vi "calibrate.vi"(8 "error in (no error)":errorcluster, 10 "device (1)":i32=1, 11 "Handle in":i64) -> (0 "error out":errorcluster, 2 "Return (<0 is error)":i32, 3 "Handle out":i64)   [LabVIEW 2016, in "OSB_uMp_library.lvlib"]
doc: "Sends calibrate command to uMp.\n\n!!! Ensure working area is clear before using this VI!!!\nuMp will move over its full range"
uses:
  OSB_uMp_library.lvlib
  ump.dll
panel:
  # "By Stuart Box at OxSyBio Ltd, 2017\n\nThis software is provided WITHOUT ANY WARRANTY; without even the implied warranty of MERCHANTABILITY or FITNESS FOR A PARTICULAR PURPOSE.\n\ninfo@oxsybio.com\n\nOxSyBio Ltd, The Walbrook Building, 25 Walbrook, London, EC4N 8AF"
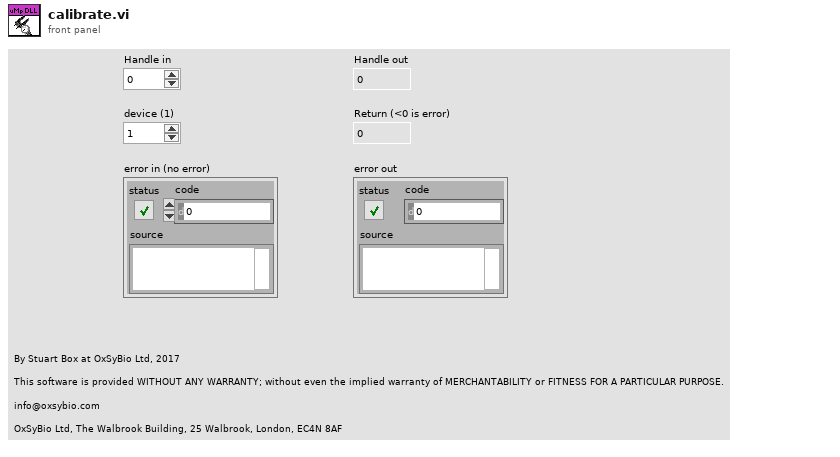
[diagram p1: front panel]
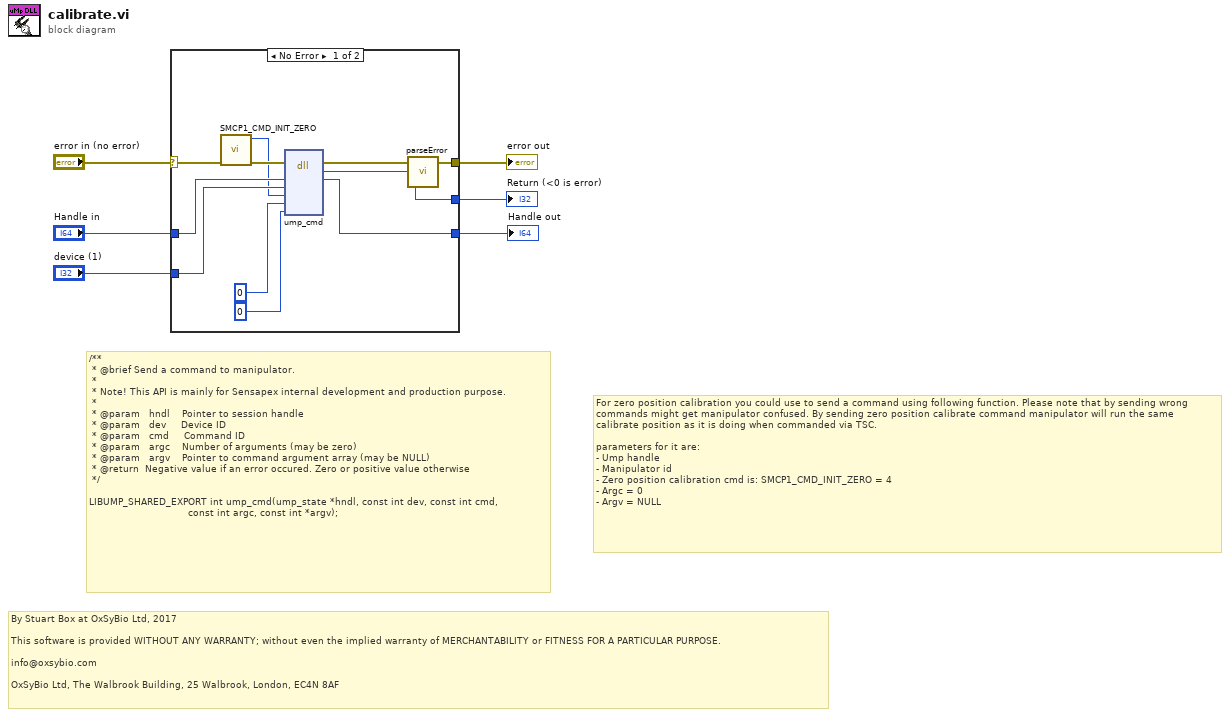
[diagram p0: block diagram]
diagram:
  # "By Stuart Box at OxSyBio Ltd, 2017\n\nThis software is provided WITHOUT ANY WARRANTY; without even the implied warranty of MERCHANTABILITY or FITNESS FOR A PARTICULAR PURPOSE.\n\ninfo@oxsybio.com\n\nOxSyBio Ltd, The Walbrook Building, 25 Walbrook, London, EC4N 8AF"
  # "For zero position calibration you could use to send a command using following function. Please note that by sending wrong commands might get manipulator confused. By sending zero position calibrate command manipulator will run the same calibrate position as it is doing when commanded via TSC.\n\nparameters for it are:\n-\tUmp handle\n-\tManipulator id\n-\tZero position calibration cmd is: SMCP1_CMD_INIT_ZERO = 4\n-\tArgc = 0\n-\tArgv = NULL"
  # "/**\n * @brief Send a command to manipulator.\n *\n * Note! This API is mainly for Sensapex internal development and production purpose.\n *\n * @param   hndl    Pointer to session handle\n * @param   dev     Device ID\n * @param   cmd     Command ID\n * @param   argc    Number of arguments (may be zero)\n * @param   argv    Pointer to command argument array (may be NULL)\n * @return  Negative value if an error occured. Zero or positive value otherwise\n */\n\nLIBUMP_SHARED_EXPORT int ump_cmd(ump_state *hndl, const int dev, const int cmd,\n                                 const int argc, const int *argv);"
  n1 = case shown="No Error" "error in (no error)" {
    selector: "error in (no error)" -> [w12 w19]
    tunnel: "Handle in" -> [w17 w18]
    tunnel: [w8 w19] -> w5
    tunnel: "device (1)" -> [w16 _]
    tunnel: [w7 _] -> w3
    tunnel: [w15 w18] -> w2
    frame No Error {
      n2 = call "SMCP1_CMD_INIT_ZERO.vi"("Error In"=w12) -> ("Error Out"=w11:errorcluster, "SMCP1_CMD_INIT_ZERO"=w10:i32)  [unwired: 9 in]
      n3 = dll-call lib="C:/Users/Stu/Desktop/OSB LabVIEW uMp/uMp_library/ump.dll" fn="ump_cmd"(error in=w11, "handle"=w17, "device"=w16, "command"=w10, "argc"=0, "argv"=0) -> (error out=w9:errorcluster, "return"=w7:i32, "handle"=w15:i64)  [unwired: 6 in, 1 out]
      n4 = call "parseError.vi"("Error In"=w9, "ump dll return value (<0 is error)"=w7) -> ("Error Out"=w8:errorcluster)  [unwired: 24 in, 1 out]
    }
    frame Error {
    }
  }
  "error out" <- w5
  "Return (<0 is error)" <- w3
  "Handle out" <- w2
